vi "CCD Acquire Spectrum with Darkcount Subtract.vi"(11 "error in":errorcluster) -> (15 "error out":errorcluster)   [LabVIEW 2020, in "Examples.lvlib"]
doc: "Example for a CCD spectrum acquisition."
uses:
  Examples.lvlib
  Classes/CCD/CCD.lvclass
  325226a6-d9db-4658-9a43-74951ce80ae1.vi
panel:
  out "XY Graph":cluster{"xAxis":dbl[], "Spectrum":dbl[]}[](graph)
  # "Connector Pane"
  # "Locals"
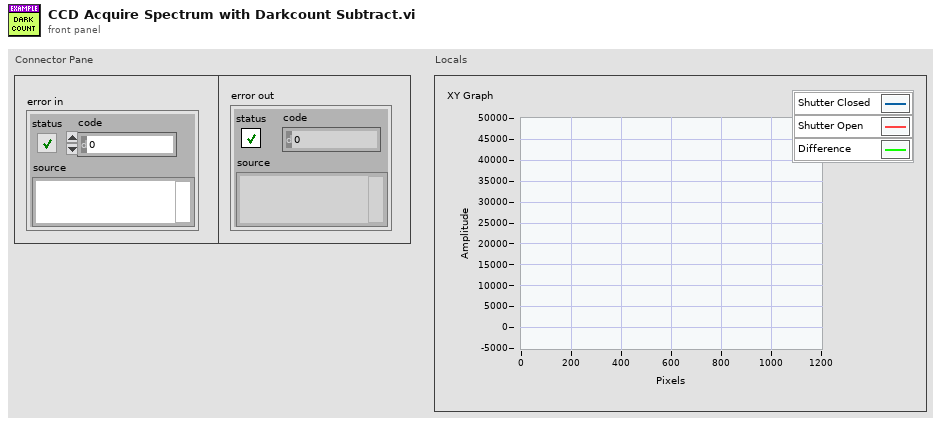
[diagram p1: front panel]
types:
  T1 = cluster{"ROI-index":i32, "xOrigin":i32, "yOrigin":i32, "xSize":i32, "ySize":i32, "xBin":i32, "yBin":i32}
  T2 = typedef "horiba.lvlib/CCD.lvclass/GetConfig.ctl" = cluster{"centerWavelength":dbl, "chipHSpacing":dbl, "chipHeight":dbl, "chipName":string, "chipSerialNumber":string, "chipVSpacing":dbl, "chipWidth":dbl, "deviceType":string, "fitParameters":dbl[], "gains":T3[], "hardwareAvgAvailable":bool, "lineScan":bool, "parallelSpeeds":T4[], "productId":string, "serialNumber":string, "signals":T5[], "speeds":T8[], "supportedFeatures":T9, "triggers":T10[], "version":string}
  T3 = typedef "horiba.lvlib/CCD.lvclass/Gain.ctl" = cluster{"info":string, "token":i32}
  T4 = typedef "horiba.lvlib/CCD.lvclass/parallelSpeed.ctl" = cluster{"info":string, "token":i32}
  T5 = typedef "horiba.lvlib/CCD.lvclass/Signal.ctl" = cluster{"events":T6[], "name":string, "token":i32}
  T6 = typedef "horiba.lvlib/CCD.lvclass/Event.ctl" = cluster{"name":string, "token":i32, "types":T7[]}
  T7 = typedef "horiba.lvlib/CCD.lvclass/Type.ctl" = cluster{"name":string, "token":i32}
  T8 = typedef "horiba.lvlib/CCD.lvclass/Speed.ctl" = cluster{"info":string, "token":i32}
  T9 = typedef "horiba.lvlib/CCD.lvclass/SupportedFeatures.ctl" = cluster{"cf_3PositionSlit":bool, "cf_CMOSOffsetCorrection":bool, "cf_Cleaning":bool, "cf_DSP":bool, "cf_DSPBin2X":bool, "cf_DelayAfterTrigger":bool, "cf_Delays":bool, "cf_EMCCD":bool, "cf_EShutter":bool, "cf_HDR":bool, "cf_Image":bool, "cf_MemorySlots":bool, "cf_Metadata":bool, "cf_MultipleExposeTimes":bool, "cf_MultipleSensors":bool, "cf_PulseSummation":bool, "cf_ROIs":bool, "cf_Signals":bool, "cf_Spectra":bool, "cf_TriggerQualifier":bool, "cf_Triggers":bool}
  T10 = typedef "horiba.lvlib/CCD.lvclass/Trigger.ctl" = cluster{"events":T6[], "name":string, "token":i32}
  T11 = typedef "horiba.lvlib/CCD.lvclass/ccdAcquisitionData.ctl" = cluster{"acqIndex":i32, "ROIs":T12[], "timestamp":string}
  T12 = typedef "horiba.lvlib/CCD.lvclass/imageAcqData.ctl" = cluster{"roiMetaData":T13, "xAxis":dbl[], "yData":dbl[][]}
  T13 = typedef "horiba.lvlib/CCD.lvclass/roiMetaData.ctl" = cluster{"roiIndex":i32, "xBinning":i32, "xOrigin":i32, "xSize":i32, "yBinning":i32, "yOrigin":i32, "ySize":i32}
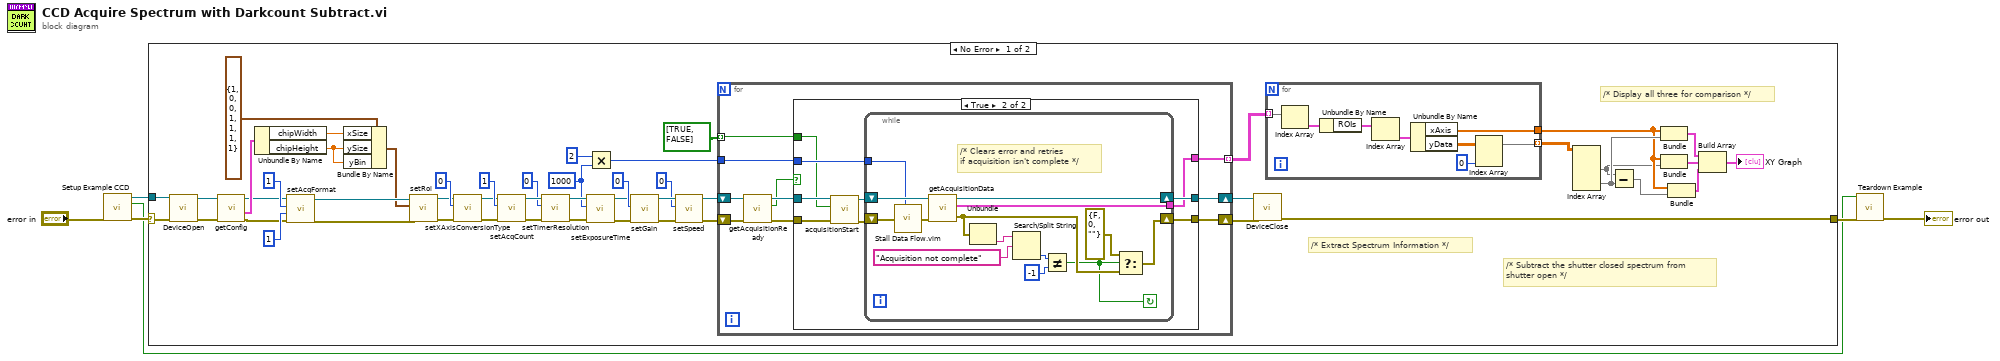
[diagram p0: block diagram]
diagram:
  n1 = call "Setup Example CCD.vi"("error in (no error)"="error in") -> ("error out"=w4:errorcluster, "Module Was Already Running?"=w1:bool, "CCD out"=w3:refnum<class "CCD.lvclass">)  [unwired: 8 in]
  n2 = case shown="No Error" w4 {
    selector: w4 -> [w57 w101]
    tunnel: w3 -> [w53 _]
    tunnel: [w55 w101] -> w2
    frame No Error {
      w18 = 1000 ("exposure time [ms] or [us]")
      # "/* Display all three for comparison */"
      # "/* Subtract the shutter closed spectrum from\nshutter open */"
      # "/* Extract Spectrum Information */"
      n3 = call-dynamic "DeviceOpen.vi"("error in (no error)"=w57, "CCD in"=w53) -> ("error out"=w13:errorcluster, "CCD out"=w12:refnum<class "CCD.lvclass">)  [unwired: 6 in, 2 out]
      n4 = call "getConfig.vi"("error in (no error)"=w13, "CCD in"=w12) -> ("error out"=w34:errorcluster, "config data"=w39:T2, "CCD out"=w35:refnum<class "CCD.lvclass">)  [unwired: 6 in, 1 out]
      n5 = Unbundle By Name(w39) -> ("chipWidth"=w15:dbl, "chipHeight"=w14:dbl)
      n6 = call "setAcqFormat.vi"("error in (no error)"=w34, "format"=1, "number of ROIs"=1, "CCD in"=w35) -> ("error out"=w41:errorcluster, "CCD out"=w40:refnum<class "CCD.lvclass">)  [unwired: 4 in, 2 out]
      n7 = Bundle By Name(cluster=T1 {"ROI-index"=1, "xOrigin"=0, "yOrigin"=0, "xSize"=1, "ySize"=1, "xBin"=1, "yBin"=1} ("roiConfig"), "xSize"=w15, "ySize"=w14, "yBin"=w14) -> (w38:T1)
      n8 = call "setRoi.vi"("error in (no error)"=w41, "roiConfig"=w38, "CCD in"=w40) -> ("error out"=w33:errorcluster, "CCD out"=w32:refnum<class "CCD.lvclass">)  [unwired: 5 in, 2 out]
      n9 = call "setXAxisConversionType.vi"("error in (no error)"=w33, "type"=0, "CCD in"=w32) -> ("error out"=w30:errorcluster, "CCD out"=w31:refnum<class "CCD.lvclass">)  [unwired: 5 in, 2 out]
      n10 = call "setAcqCount.vi"("error in (no error)"=w30, "count"=1, "CCD in"=w31) -> ("error out"=w28:errorcluster, "CCD out"=w29:refnum<class "CCD.lvclass">)  [unwired: 5 in, 2 out]
      n11 = call "setTimerResolution.vi"("error in (no error)"=w28, "resolutionToken"=0, "CCD in"=w29) -> ("error out"=w26:errorcluster, "CCD out"=w27:refnum<class "CCD.lvclass">)  [unwired: 5 in, 2 out]
      n12 = call "setExposureTime.vi"("error in (no error)"=w26, "exposure time [ms] or [us]"=w18, "CCD in"=w27) -> ("error out"=w21:errorcluster, "CCD out"=w20:refnum<class "CCD.lvclass">)  [unwired: 5 in, 2 out]
      n13 = Multiply(x=2, y=w18) -> (x*y=w9:i32)
      n14 = call "setGain.vi"("error in (no error)"=w21, "token"=0, "CCD in"=w20) -> ("error out"=w24:errorcluster, "CCD out"=w25:refnum<class "CCD.lvclass">)  [unwired: 5 in, 2 out]
      n15 = call "setSpeed.vi"("error in (no error)"=w24, "token"=0, "CCD in"=w25) -> ("error out"=w11:errorcluster, "CCD out"=w10:refnum<class "CCD.lvclass">)  [unwired: 5 in, 2 out]
      n16 = for {
        tunnel: [w60] -> w7 mode=indexing
        tunnel: bool[] [TRUE, FALSE] ("openShutter") -> [w62] mode=indexing
        shift-right: [w58] -> w56
        shift-left: w11 -> [w64]
        shift-right: [w59] -> w54
        shift-left: w10 -> [w63]
        tunnel: w9 -> [w61]
        n17 = call "getAcquisitionReady.vi"("error in (no error)"=w64, "CCD in"=w63) -> ("error out"=w67:errorcluster, "ready"=w65:bool, "CCD out"=w66:refnum<class "CCD.lvclass">)  [unwired: 7 in]
        n18 = case shown="True" w65 {
          tunnel: w67 -> [w68 w78]
          tunnel: w66 -> [w69 w77]
          tunnel: [w68 w73] -> w58
          tunnel: [w69 w74] -> w59
          tunnel: [_ w71] -> w60
          tunnel: w61 -> [_ w72]
          tunnel: w62 -> [_ w70]
          frame False {
          }
          frame True {
            n19 = call "acquisitionStart.vi"("error in (no error)"=w78, "openShutter"=w70, "CCD in"=w77) -> ("error out"=w75:errorcluster, "CCD out"=w76:refnum<class "CCD.lvclass">)  [unwired: 5 in, 2 out]
            n20 = while {
              shift-right: [w91] -> w74
              shift-left: w76 -> [w92]
              tunnel: [w90] -> w71
              shift-right: [w80] -> w73
              shift-left: w75 -> [w87]
              tunnel: w72 -> [w89]
              stop <- w79 continue-if-true
              # "/* Clears error and retries\nif acquisition isn't complete */"
              n21 = call "Stall Data Flow.vim"("value in"=w87, "milliseconds to wait"=w89) -> ("value out"=w88:errorcluster)  [unwired: 1 out]
              n22 = call "getAcquisitionData.vi"("error in (no error)"=w88, "CCD in"=w92) -> ("error out"=w81:errorcluster, "ccdAcquisitions"=w90:T11[], "CCD out"=w91:refnum<class "CCD.lvclass">)  [unwired: 6 in, 1 out]
              n23 = Unbundle(w81) -> ("source"=w85:string)  [unwired: 2 out]
              n24 = Search/Split String(string=w85, search string/char (-)="Acquisition not complete") -> (offset of match=w84:i32)  [unwired: 1 in, 2 out]
              n25 = Not Equal?(x=w84, y=-1) -> (x != y?=w79:bool)
              n26 = Select(t=errorcluster {"status"=FALSE, "code"=0, "source"=""} ("error out"), s=w79, f=w81) -> (s? t:f=w80:errorcluster)
            }
          }
        }
      }
      n27 = call-dynamic "DeviceClose.vi"("error in (no error)"=w56, "CCD in"=w54) -> ("error out"=w55:errorcluster)  [unwired: 5 in, 4 out]
      n28 = for {
        tunnel: w7 -> [w100] mode=indexing
        tunnel: [w96] -> w49
        tunnel: [w94] -> w52 mode=indexing
        n29 = Index Array(array=w100) -> (element=w99:T11)  [unwired: 1 in]
        n30 = Unbundle By Name(w99) -> ("ROIs"=w98:T12[])
        n31 = Index Array(array=w98) -> (element=w97:T12)  [unwired: 1 in]
        n32 = Unbundle By Name(w97) -> ("xAxis"=w96:dbl[], "yData"=w95:dbl[][])
        n33 = Index Array(array=w95, index (col)=0 ("disabled index (col)")) -> (element=w94:dbl[])  [unwired: 1 in]
      }
      n34 = Index Array(array=w52) -> (element #1=w48:dbl[], element #2=w50:dbl[])  [unwired: 4 in]
      n35 = Subtract(x=w48, y=w50) -> (x-y=w51:dbl[])
      n36 = Bundle("xAxis"=w49, "yData"=w50) -> (w47:cluster{"xAxis":dbl[], "yData":dbl[]})  [unwired: 1 in]
      n37 = Bundle("xAxis"=w49, "yData"=w48) -> (w46:cluster{"xAxis":dbl[], "yData":dbl[]})  [unwired: 1 in]
      n38 = Bundle("xAxis"=w49, w51) -> (w45:cluster{"xAxis":dbl[], dbl[]})  [unwired: 1 in]
      n39 = Build Array(w47, w46, w45) -> (→"XY Graph":cluster{"xAxis":dbl[], "yData":dbl[]}[])
    }
    frame Error {
    }
  }
  n40 = call "Teardown Example.vi"("error in (no error)"=w2, "Module Was Already Running?"=w1) -> ("error out"=→"error out":errorcluster)  [unwired: 9 in]
